vi "DriveExecute.vi"(8 "error in (no error)":errorcluster) -> (0 "error out":errorcluster)   [LabVIEW 2020]
doc: "Execute for Drie\n\nClosed control loop for drive\n\ninput: \n error in (cluster)\n\noutput:\n error out (cluster)"
uses:
  <vilib>/Rock Robotics/WPI/ThirdParty/JAS_Junk/TrajLib/LinearFilter_ResetToValue.vi
  <vilib>/Rock Robotics/WPI/ThirdParty/JAS_Junk/TrajLib/LinearFilter_Calculate.vi
  DriveGlobal.vi
  <vilib>/Rock Robotics/WPI/ThirdParty/JAS_Junk/TrajLib/LinearFilter_MovingAverage.vi
  <vilib>/Rock Robotics/WPI/ThirdParty/JAS_Junk/TrajLib/LinearFilter_LowPassBW1.vi
  <vilib>/Rock Robotics/WPI/ThirdParty/JAS_Junk/TrajLib/LinearFilter_LowPassBW2.vi
  <vilib>/Rock Robotics/WPI/ThirdParty/JAS_Junk/TrajLib/LinearFilter_HighPassBW1.vi
  <vilib>/Rock Robotics/WPI/ThirdParty/JAS_Junk/TrajLib/LinearFilter_HighPassBW2.vi
  <vilib>/Rock Robotics/WPI/ThirdParty/JAS_Junk/TrajLib/Trajectory_Library.lvlib
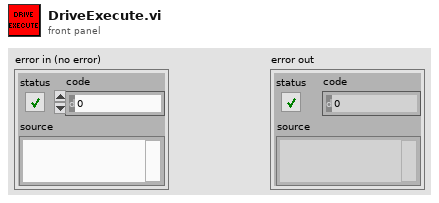
[diagram p1: front panel]
types:
  T1 = enum16{"Moving Average", "Low Pass 1st Order Butterworth", "Low Pass 2nd Order Butterworth", "High Pass 1st Order Butterworth", "High Pass 2nd Order Butterworth"}
  T2 = typedef "ADIS16470 Device Reference.ctl" = cluster{"DevStatus":errorcluster, "Hardware Config":T3, "Calibration Complete":refnum<notifier>, "Status Reference":refnum<data-value>, "Data Reference":refnum<data-value>, "Sychronous Process VI":T7, "Cmd FIFO":refnum<k33>, "Source":T8, "Data FIFO":refnum<k33>, "Calibration Time (ms)":u32, "Data Reference":refnum<data-value>}
  T3 = typedef "ADIS16470 Hardware Configuration.ctl" = cluster{"SPI Clock Rate (Hz)":dbl, "IMU SPI Mode (3)":T4, "IMU Reset Pin":T5, "IMU SPI Bus":T6, "IMU Data Ready Pin":T5, "Stall Config":cluster{"Pow2BytesPerRead":u8, "StallTicks":u16, "CsToSclkTicks":u8}}
  T4 = typedef "WPI_SPIMode.ctl" = enum16{"Mode 0 (Clk Idle Low,Sample on Leading)", "Mode 1 (Clk Idle Low,Sample on Trailing)", "Mode 2 (Clk Idle High,Sample on Leading)", "Mode 3 (Clk Idle High,Sample on Trailing)"}
  T5 = typedef "FPGA_DIOChannel.ctl" = enum8{"DIO 0", "DIO 1", "DIO 2", "DIO 3", "DIO 4", "DIO 5", "DIO 6", "DIO 7", "DIO 8", "DIO 9", "DIO MXP 0", "DIO MXP 1", "DIO MXP 2", "DIO MXP 3", "DIO MXP 4", "DIO MXP 5", "DIO MXP 6", "DIO MXP 7", "DIO MXP 8", "DIO MXP 9", "DIO MXP 10", "DIO MXP 11", "DIO MXP 12", "DIO MXP 13", "DIO MXP 14", "DIO MXP 15", "SPI Port CS1", "SPI Port CS2", "SPI Port CS3", "SPI Port MISO", "SPI Port MOSI", "Invalid"}
  T6 = typedef "spi_bus.ctl" = enum16{"SPI On-Board, CS0", "SPI On-Board, CS1", "SPI On-Board, CS2", "SPI On-Board, CS3", "SPI MXP", "Invalid"}
  T7 = typedef "ADIS16470 Process.ctl" = refnum<vi>
  T8 = typedef "FPGA_CounterEncoderSourceConvertionLVSourceType.ctl" = cluster{"DevStatus":errorcluster, "AnalogTriggerMode?":bool, "DigitalMode":cluster{"DIO Channel":T9}, "AnalogTriggerMode":cluster{"AnalogTriggerIndex":T10, "OutputType":T11}}
  T9 = typedef "FPGA_DIODigitalSourceChannel.ctl" = enum8{"DIO 0", "DIO 1", "DIO 2", "DIO 3", "DIO 4", "DIO 5", "DIO 6", "DIO 7", "DIO 8", "DIO 9", "DIO MXP 0", "DIO MXP 1", "DIO MXP 2", "DIO MXP 3", "DIO MXP 4", "DIO MXP 5", "DIO MXP 6", "DIO MXP 7", "DIO MXP 8", "DIO MXP 9", "DIO MXP 10", "DIO MXP 11", "DIO MXP 12", "DIO MXP 13", "DIO MXP 14", "DIO MXP 15", "SPI Port CS1", "SPI Port CS2", "SPI Port CS3", "SPI Port MISO", "SPI Port MOSI", "Disabled"}
  T10 = typedef "FPGA_AnalogTriggerIndex.ctl" = enum8{"Trig 0", "Trig 1", "Trig 2", "Trig 3", "Trig 4", "Trig 5", "Trig 6", "Trig 7", "Invalid"}
  T11 = typedef "FPGA_AnalogTriggerOutType.ctl" = enum16{"InWindow", "TriggerState", "Rising", "Falling"}
  T12 = typedef "Trajectory_Library.lvlib/SWERVE_DRIVE_KINEMATICS.ctl" = cluster{"NumModules":i32, "InverseKinematics":T13, "ForwardKinematics":T13, "Modules":T14[], "PrevCoR":T14, "SavedModuleStates":T15[]}
  T13 = typedef "NI_Matrix.lvlib/RealMatrix.ctl" = dbl[][]
  T14 = typedef "Trajectory_Library.lvlib/TRANSLATION2D.ctl" = cluster{"X":dbl, "Y":dbl}
  T15 = typedef "Trajectory_Library.lvlib/SWERVE_DRIVE_MODULE_STATE.ctl" = cluster{"Speed":dbl, "Angle":T16}
  T16 = typedef "Trajectory_Library.lvlib/ROTATION2D.ctl" = cluster{"VALUE":dbl, "COS":dbl, "SIN":dbl}
  T17 = typedef "ADIS16470 Status.ctl" = cluster{"Calibrated?":bool, "IMU Detected?":bool}
  T18 = typedef "Trajectory_Library.lvlib/SWERVE_DRIVE_MODULE_POSITION.ctl" = cluster{"Distance":dbl, "Angle":T16, "P":bool}
  T19 = typedef "Trajectory_Library.lvlib/CHASSIS_SPEEDS.ctl" = cluster{"vX":dbl, "vY":dbl, "vOmega":dbl}
  T20 = typedef "ADIS16470 Data.ctl" = cluster{"XAngle":dbl, "YAngle":dbl, "ZAngle":dbl}
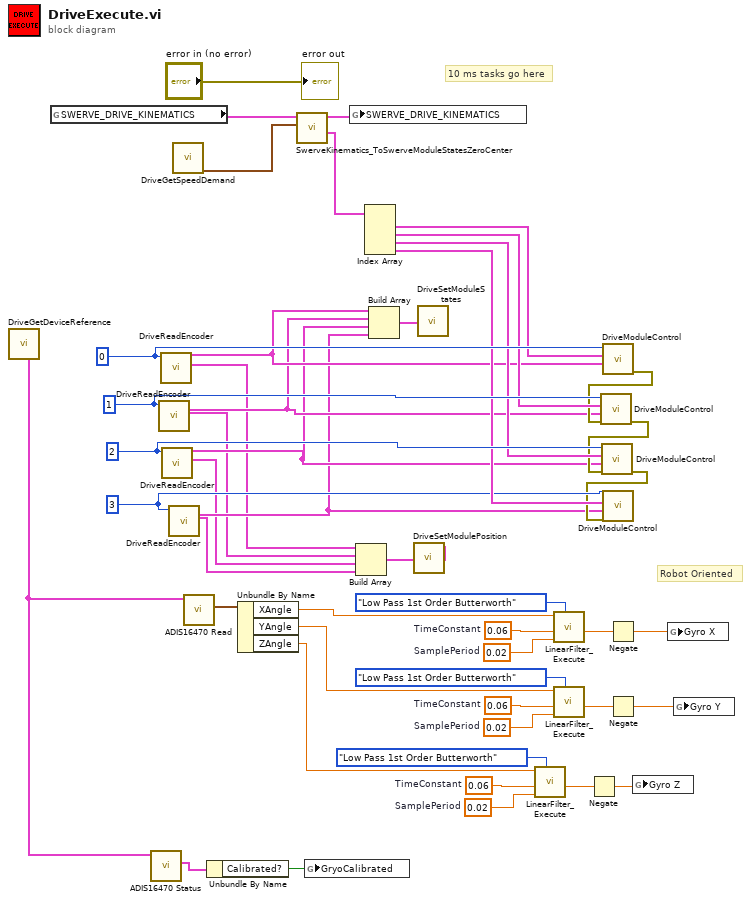
[diagram p0: block diagram]
diagram:
  w22 = 0 ("ModualNamePrefix")
  w21 = 1 ("ModualNamePrefix")
  w20 = 2 ("ModualNamePrefix")
  w14 = 3 ("ModualNamePrefix")
  w31 = 0.02  # SamplePeriod
  w30 = 0.06  # TimeConstant
  w37 = 0.02  # SamplePeriod
  w36 = 0.06  # TimeConstant
  w42 = 0.02  # SamplePeriod
  w41 = 0.06  # TimeConstant
  # "Robot Oriented"
  # "10 ms tasks go here"
  n1 = call "DriveGetDeviceReference.vi"() -> ("Gryo"=w43:T2)  [unwired: 11 in]
  n2 = global read "DriveGlobal.vi" "SWERVE_DRIVE_KINEMATICS"() -> (w25:T12)
  n3 = call <vilib>:"ADIS16470 Status.vi"("ADIS16470DevRef"=w43) -> ("ADIS16470 Status"=w45:T17)  [unwired: 8 in, 2 out]
  n4 = call "DriveReadEncoder.vi"("ModualNamePrefix"=w21) -> ("SWERVE_DRIVE_MODULE_POSITION"=w6:T18, "SWERVE_DRIVE_MODULE_STATE"=w9:T15)  [unwired: 9 in]
  n5 = call "DriveReadEncoder.vi"("ModualNamePrefix"=w22) -> ("SWERVE_DRIVE_MODULE_POSITION"=w3:T18, "SWERVE_DRIVE_MODULE_STATE"=w10:T15)  [unwired: 9 in]
  n6 = call "DriveReadEncoder.vi"("ModualNamePrefix"=w20) -> ("SWERVE_DRIVE_MODULE_POSITION"=w5:T18, "SWERVE_DRIVE_MODULE_STATE"=w8:T15)  [unwired: 9 in]
  n7 = call "DriveReadEncoder.vi"("ModualNamePrefix"=w14) -> ("SWERVE_DRIVE_MODULE_POSITION"=w4:T18, "SWERVE_DRIVE_MODULE_STATE"=w7:T15)  [unwired: 9 in]
  n8 = call "DriveGetSpeedDemand.vi"() -> ("ChassisSpeedDemand"=w24:T19)  [unwired: 8 in, 3 out]
  n9 = call <vilib>:"ADIS16470 Read.vi"("ADIS16470DevRef"=w43) -> ("ADIS16470 Value"=w47:T20)  [unwired: 7 in, 3 out]
  n10 = Unbundle By Name(w45) -> ("Calibrated?"=w44:bool)
  n11 = Unbundle By Name(w47) -> ("XAngle"=w26:dbl, "YAngle"=w33:dbl, "ZAngle"=w39:dbl)
  n12 = call <vilib>:"SwerveKinematics_ToSwerveModuleStatesZeroCenter.vi"("ChassisSpeeds"=w24, "in SWERVE_DRIVE_KINEMATICS"=w25) -> ("ModuleStates"=w19:T15[], "out SWERVE_DRIVE_KINEMATICS"=w23:T12)  [unwired: 8 in]
  n13 = global write "DriveGlobal.vi" "GryoCalibrated"(w44) -> ()
  n14 = global write "DriveGlobal.vi" "SWERVE_DRIVE_KINEMATICS"(w23) -> ()
  n15 = Build Array(w3, w6, w5, w4) -> (w2:T18[])
  n16 = Index Array(array=w19) -> (element #1=w15:T15, element #2=w18:T15, element #3=w17:T15, element #4=w16:T15)  [unwired: 4 in]
  n17 = Build Array(w10, w9, w8, w7) -> (w1:T15[])
  n18 = call "DriveSetModulePosition.vi"("ModulePosition"=w2) -> ()  [unwired: 11 in]
  n19 = call "DriveSetModuleStates.vi"("ModuleStates"=w1) -> ()  [unwired: 11 in]
  n20 = call <vilib>:"LinearFilter_Execute.vi"("Filter Type"=T1."Low Pass 1st Order Butterworth", "SamplePeriod"=w42, "TimeConstant"=w41, "Input"=w39) -> ("Output"=w38:dbl)  [unwired: 6 in, 1 out]
  n21 = call <vilib>:"LinearFilter_Execute.vi"("Filter Type"=T1."Low Pass 1st Order Butterworth", "SamplePeriod"=w31, "TimeConstant"=w30, "Input"=w26) -> ("Output"=w28:dbl)  [unwired: 6 in, 1 out]
  n22 = call <vilib>:"LinearFilter_Execute.vi"("Filter Type"=T1."Low Pass 1st Order Butterworth", "SamplePeriod"=w37, "TimeConstant"=w36, "Input"=w33) -> ("Output"=w34:dbl)  [unwired: 6 in, 1 out]
  n23 = Negate(x=w38) -> (-x=w46:dbl)
  n24 = call "DriveModuleControl.vi"("Actual State"=w10, "Desired State"=w15, "ModualNamePrefix"=w22) -> ("error out"=w13:errorcluster)  [unwired: 8 in]
  n25 = call "DriveModuleControl.vi"("error in"=w13, "Actual State"=w9, "Desired State"=w18, "ModualNamePrefix"=w21) -> ("error out"=w12:errorcluster)  [unwired: 7 in]
  n26 = call "DriveModuleControl.vi"("error in"=w12, "Actual State"=w8, "Desired State"=w17, "ModualNamePrefix"=w20) -> ("error out"=w11:errorcluster)  [unwired: 7 in]
  n27 = call "DriveModuleControl.vi"("error in"=w11, "Actual State"=w7, "Desired State"=w16, "ModualNamePrefix"=w14) -> ()  [unwired: 7 in, 1 out]
  n28 = Negate(x=w28) -> (-x=w27:dbl)
  n29 = Negate(x=w34) -> (-x=w32:dbl)
  n30 = global write "DriveGlobal.vi" "Gyro Z"(w46) -> ()
  n31 = global write "DriveGlobal.vi" "Gyro X"(w27) -> ()
  n32 = global write "DriveGlobal.vi" "Gyro Y"(w32) -> ()
  "error out" <- "error in (no error)"
